vi "Draw_Rect_Text.vi"(5 "Rotation":dbl format="%#_13g", 6 "Color":u32(colorbox)=16711680, 7 "ROI?":bool, 8 "error in (no error)":errorcluster, 9 "RIO Input":T2 {"Contours"."Type" items=["No Selection", "Point", "Line", "Rectangle", "Oval", "Polygon", "Freehand Region", "Annulus", "Unused2", "Unused3", "Broken Line", "Freehand Line", "Rotated Rectangle"]}, 10 "Bounding Box":cluster{"x":sgl, "y":sgl}[](array[cluster]), 11 "Image":T1) -> (0 "error out":errorcluster, 3 "Image 2":T1)   [LabVIEW 2017]
uses:
  <vilib>/vision/Image Controls.llb/IMAQ Image.ctl
panel:
  out "error out 2":errorcluster
  in  "Drawing Mode (Frame)":u32(ring) items=["Frame", "Fill", "Highlight"]
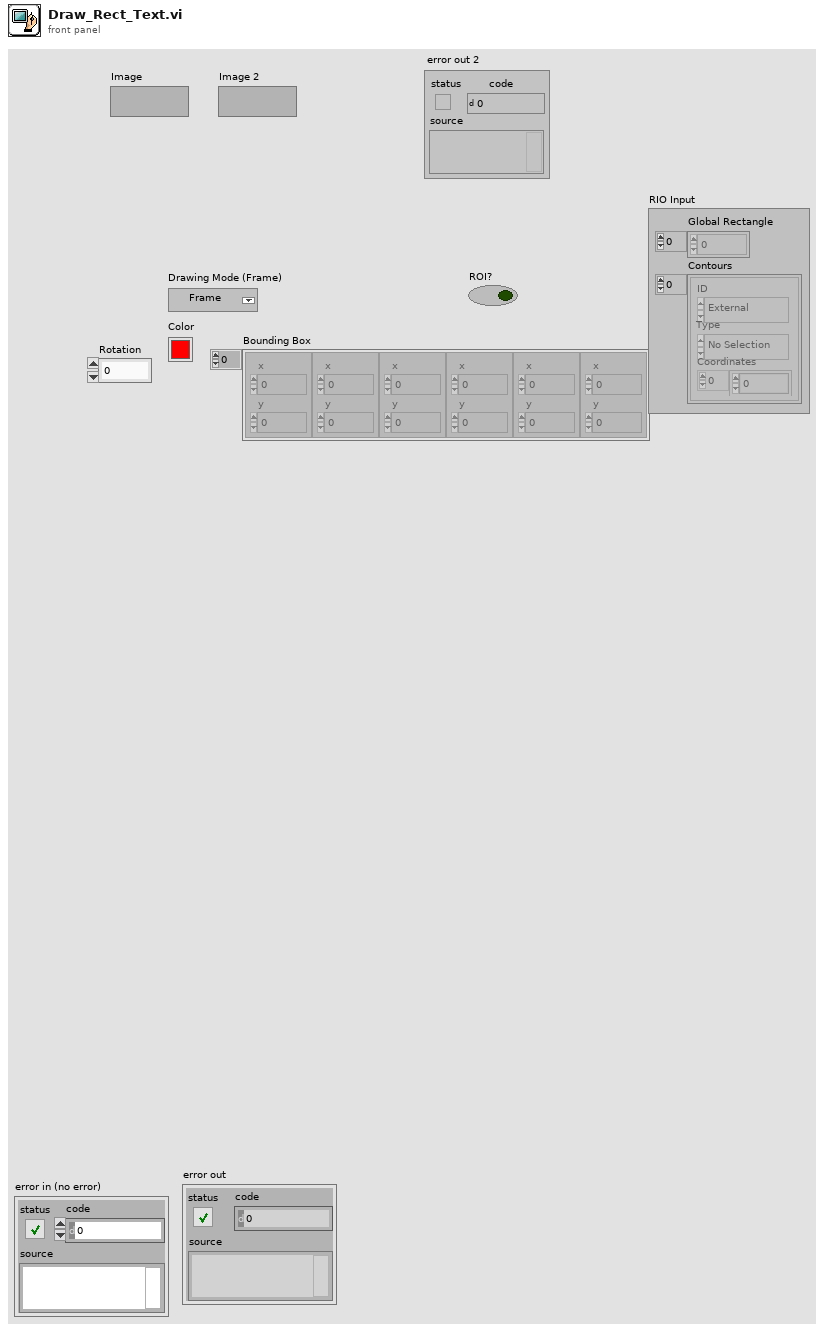
[diagram p1: front panel]
types:
  T1 = typedef "IMAQ Image.ctl" = refnum<image>
  T2 = typedef "ROI Descriptor" = cluster{"Global Rectangle":i32[], "Contours":cluster{"ID":enum32{"External", "Internal"}, "Type":u32, "Coordinates":i32[]}[]}
  T3 = typedef "IMAQ Rectangle" = cluster{"Left":i32, "Top":i32, "Right":i32, "Bottom":i32, "Rotation":dbl}
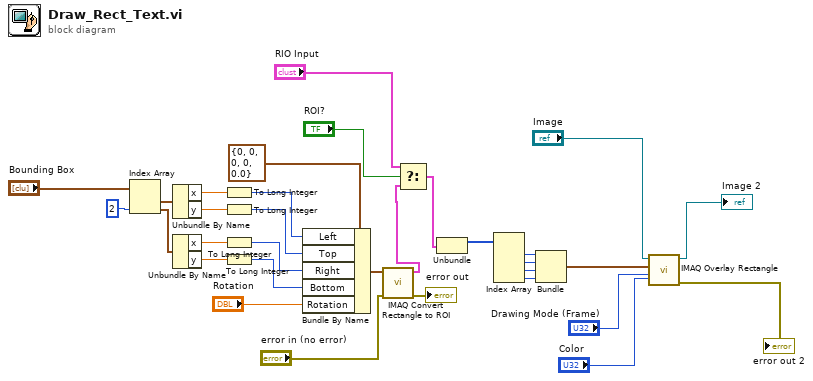
[diagram p0: block diagram]
diagram:
  n1 = Index Array(array="Bounding Box", index #2=2 ("index")) -> (element #1=w20:cluster{"x":sgl, "y":sgl}, element #2=w21:cluster{"x":sgl, "y":sgl})  [unwired: 1 in]
  n2 = Unbundle By Name(w20) -> ("x"=w25:sgl, "y"=w26:sgl)
  n3 = Unbundle By Name(w21) -> ("x"=w27:sgl, "y"=w28:sgl)
  n4 = To Long Integer(number=w25) -> (32bit integer=w29:i32)
  n5 = To Long Integer(number=w26) -> (32bit integer=w30:i32)
  n6 = To Long Integer(number=w27) -> (32bit integer=w31:i32)
  n7 = To Long Integer(number=w28) -> (32bit integer=w32:i32)
  n8 = Bundle By Name(cluster=T3 {"Left"=0, "Top"=0, "Right"=0, "Bottom"=0, "Rotation"=0.0} ("Rectangle"), "Left"=w29, "Top"=w30, "Right"=w31, "Bottom"=w32, "Rotation"="Rotation") -> (w22:T3)
  n9 = call "IMAQ Convert Rectangle to ROI"("error in (no error)"="error in (no error)", "Rectangle"=w22) -> ("error out"=→"error out":errorcluster, "ROI Descriptor"=w9:T2)  [unwired: 7 in]
  n10 = Select(t="RIO Input", s="ROI?", f=w9) -> (s? t:f=w10:T2)
  n11 = Unbundle(w10) -> ("Global Rectangle"=w17:i32[])  [unwired: 1 out]
  n12 = Index Array(array=w17) -> (element #1=w15:i32, element #2=w14:i32, element #3=w13:i32, element #4=w16:i32)  [unwired: 4 in]
  n13 = Bundle(w15, w14, w13, w16) -> (w6:cluster{i32, i32, i32, i32})  [unwired: 1 in]
  n14 = call "IMAQ Overlay Rectangle"("Color"="Color", "Drawing Mode (Frame)"="Drawing Mode (Frame)", "Rectangle"=w6, "Image"="Image") -> ("error out"=→"error out 2":errorcluster, "Image Out"=→"Image 2":T1)  [unwired: 6 in]
